vi "ziModSetValueDoubleArray.vi"(8 "Error In":errorcluster, 9 "Values":dbl[](array[numeric]), 10 "Paths":string[](array[string]), 11 "ModHandle In":T1 {"ModHandle" format="0x%08x"; "Conn" format="0x%08x"}) -> (0 "Error Out":errorcluster, 3 "ModHandle Out":T1 {"ModHandle" format="0x%08x"; "Conn" format="0x%08x"})   [LabVIEW 2018, in "Zurich Instruments LabOne.lvlib"]
doc: "This vi sets values of the specified <b>module </b> nodes in <b>Path</b> to <b>Value</b>., e.g sweep/endless"
uses:
  Zurich Instruments LabOne.lvlib
  ziTypeModHandle.ctl
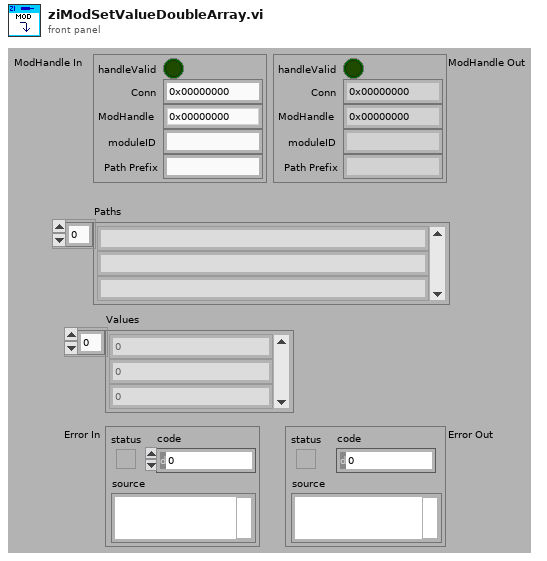
[diagram p1: front panel]
types:
  T1 = typedef "Zurich Instruments LabOne.lvlib/ziTypeModHandle.ctl" = cluster{"handleValid":bool, "Conn":u64, "ModHandle":u64, "moduleID":string, "Path Prefix":string}
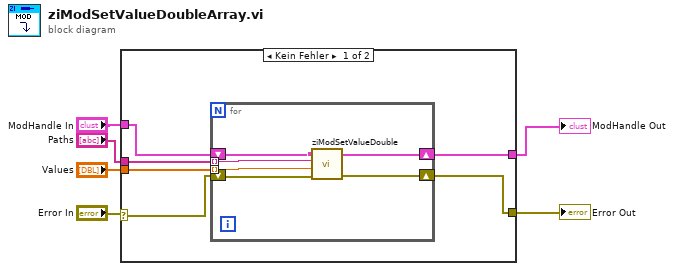
[diagram p0: block diagram]
diagram:
  n1 = case shown="Kein Fehler" "Error In" {
    selector: "Error In" -> [w9 w20]
    tunnel: [w10 w20] -> w6
    tunnel: "ModHandle In" -> [w12 w19]
    tunnel: [w11 w19] -> w3
    tunnel: "Values" -> [w8 _]
    tunnel: "Paths" -> [w7 _]
    frame No Error {
      n2 = for {
        tunnel: w7 -> [w18] mode=indexing
        tunnel: w8 -> [w17] mode=indexing
        shift-right: [w15] -> w10
        shift-left: w9 -> [w16]
        shift-right: [w14] -> w11
        shift-left: w12 -> [w13]
        n3 = call "ziModSetValueDouble.vi"("Error In"=w16, "Value"=w17, "Path"=w18, "ModHandle In"=w13) -> ("Error Out"=w15:errorcluster, "ModHandle Out"=w14:T1)  [unwired: 6 in]
      }
    }
    frame Error {
    }
  }
  "Error Out" <- w6
  "ModHandle Out" <- w3
